vi "bars.vi"() -> ()   [LabVIEW 2015]
panel:
  out "Numeric 4":i32
  out "Rejected 2":i32(slide) scale=0.0..20.0
  out "Numeric 5":i32
  out "Pending 2":i32(slide) scale=0.0..20.0
  out "Numeric 6":i32
  out "Acepted 2":i32(slide) scale=0.0..1000.0
  out "Numeric 3":i32
  out "Numeric 2":i32
  out "Numeric":i32
  out "Acepted":i32(slide) scale=0.0..1000.0
  out "Rejected":i32(slide) scale=0.0..20.0
  out "Pending":i32(slide) scale=0.0..20.0
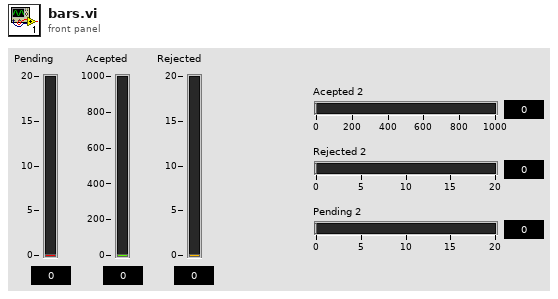
[diagram p1: front panel]
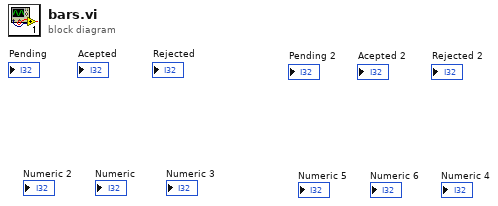
[diagram p0: block diagram]
diagram:
